vi "Calibration-file-maker.vi"() -> ()   [LabVIEW 2021]
uses:
  <vilib>/Utility/file.llb/Write Delimited Spreadsheet (DBL).vi
panel:
  in  "Error":dbl
  in  "Number of points":i32
  in  "Max":dbl
  in  "Min":dbl
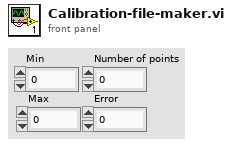
[diagram p1: front panel]
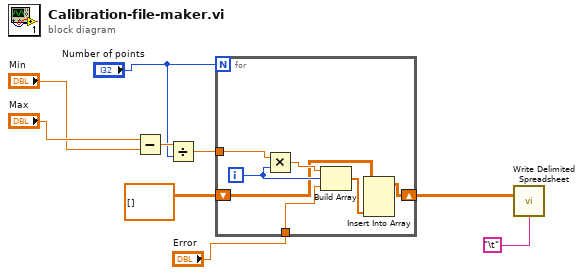
[diagram p0: block diagram]
diagram:
  n1 = Subtract(x="Max", y="Min") -> (x-y=w7:dbl)
  n2 = Divide(x=w7, y="Number of points") -> (x/y=w5:dbl)
  n3 = for {
    N: "Number of points" -> [_]
    tunnel: w5 -> [w16]
    shift-right: [w10] -> w2
    shift-left: dbl[][] [] ("array") -> [w12]
    tunnel: "Error" -> [w13]
    i -> [w14]
    n4 = Multiply(x=w16, y=w14) -> (x*y=w15:dbl)
    n5 = Build Array(w15, w14, w13) -> (w11:dbl[])
    n6 = Insert Into Array(array=w12, new element=w11) -> (w10:dbl[][])  [unwired: 2 in]
  }
  n7 = call-poly <vilib>:"Write Delimited Spreadsheet.vi"("2D data"=w2, "delimiter (\\t)"="\t") -> ()  [unwired: 12 in, 2 out]
